vi "Day 18-Get Magnitude.vi"(11 "Array in":i32[][](array[numeric])) -> (3 "Magnitude":i32)   [LabVIEW 2021]
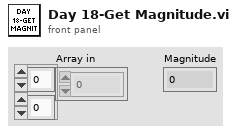
[diagram p1: front panel]
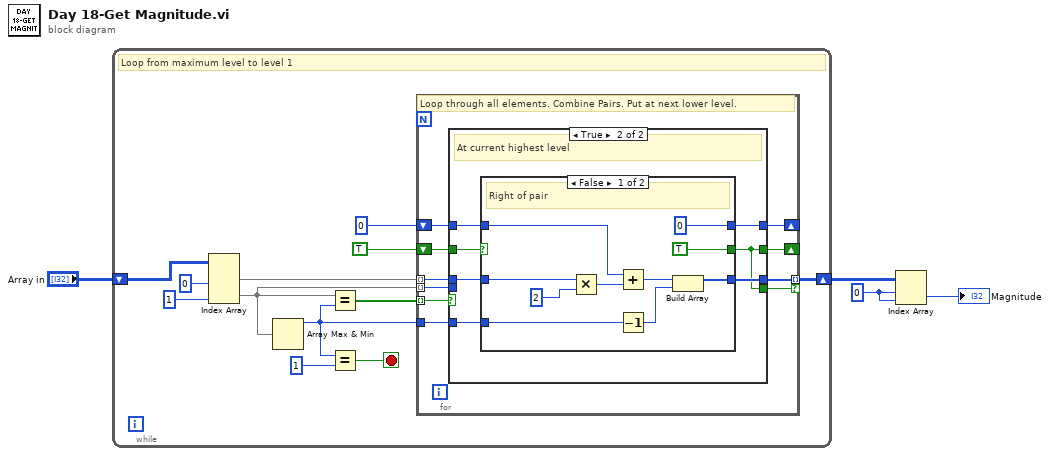
[diagram p0: block diagram]
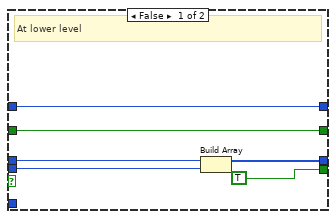
[diagram p2: hidden frame]
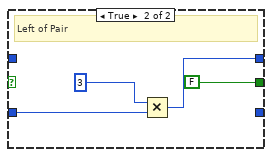
[diagram p3: hidden frame]
diagram:
  w3 = 0 ("index (row)")
  n1 = while {
    shift-right: [w9] -> w2
    shift-left: "Array in" -> [w14]
    stop <- w6 stop-if-true
    # "Loop from maximum level to level 1"
    n2 = Index Array(array=w14, index (col) #1=0 ("disabled index (col)"), index (col) #2=1 ("disabled index (col)")) -> (element #1=w12:i32[], element #2=w5:i32[])  [unwired: 2 in]
    n3 = Array Max & Min(array=w5) -> (max value=w8:i32)  [unwired: 3 out]
    n4 = Equal?(x=w5, y=w8) -> (x = y?=w15:bool[])
    n5 = Equal?(x=w8, y=1) -> (x = y?=w6:bool)
    n6 = for {
      tunnel: w15 -> [w26] mode=indexing
      tunnel: w12 -> [w25] mode=indexing
      shift-right: [w21] -> _
      shift-left: TRUE -> [w24]
      shift-right: [w23] -> _
      shift-left: 0 -> [w22]
      tunnel: w8 -> [w20]
      tunnel: [w19] -> w9 mode=indexing if=w18
      tunnel: w5 -> [w17] mode=indexing
      # "Loop through all elements. Combine Pairs. Put at next lower level."
      n7 = case shown="True" w26 {
        tunnel: w25 -> [w31 w39]
        tunnel: w24 -> [w32 w38]
        tunnel: [w28 w36] -> w23
        tunnel: w22 -> [w28 w37]
        tunnel: [w32 w33] -> w21
        tunnel: w20 -> [_ w35]
        tunnel: [w30 w34] -> w19
        tunnel: [TRUE w33] -> w18
        tunnel: w17 -> [w27 _]
        frame False {
          # "At lower level"
          n8 = Build Array(w31, w27) -> (w30:i32[])
        }
        frame True {
          # "At current highest level"
          n9 = case shown="False" w38 {
            tunnel: w39 -> [w48 w53]
            tunnel: [TRUE FALSE] -> w33
            tunnel: w37 -> [w44 _]
            tunnel: [0 w50] -> w36
            tunnel: w35 -> [w42 _]
            tunnel: [w40 _] -> w34
            frame False {
              # "Right of pair"
              n10 = Multiply(x=w48, y=2) -> (x*y=w45:i32)
              n11 = Add(x=w44, y=w45) -> (x+y=w43:i32)
              n12 = Decrement(x=w42) -> (x-1=w41:i32)
              n13 = Build Array(w43, w41) -> (w40:i32[])
            }
            frame True {
              # "Left of Pair"
              n14 = Multiply(x=3, y=w53) -> (x*y=w50:i32)
            }
          }
        }
      }
    }
  }
  n15 = Index Array(array=w2, index (row)=w3, index (col)=w3) -> (element=→"Magnitude":i32)
